vi "Chroma3.0.vi"() -> ()   [LabVIEW 2015]
uses:
  <vilib>/Utility/file.llb/Write To Spreadsheet File (string).vi
panel:
  in  "Run Name":string
  in  "Type (V_THD)":u32(ring) caption="Type (V_RMS)" items=["V_THD"=3, "V_PEAK-"=2, "V_RMS"=0, "V_PEAK+"=1]
  in  "Type (I_THD)":u32(ring) caption="Type (I_RMS)" items=["I_RMS"=0, "I_PEAK-"=2, "I_INRUSH"=3, "I_CRESTFACTOR"=4, "I_THD"=5, "I_PEAK+"=1]
  in  "Type (V_PEAK+)":u32(ring) caption="Type (V_RMS)" items=["V_THD"=3, "V_PEAK-"=2, "V_RMS"=0, "V_PEAK+"=1]
  in  "Type (P_FACTOR)":u32(ring) caption="Type (P_REAL)" items=["P_REAL"=0, "P_APPARENT"=1, "P_REACTIVE"=2, "P_ENERGY"=4, "P_FACTOR"=3]
  in  "Type (P_REACTIVE)":u32(ring) caption="Type (P_REAL)" items=["P_REAL"=0, "P_APPARENT"=1, "P_FACTOR"=3, "P_ENERGY"=4, "P_REACTIVE"=2]
  in  "Type (P_APPARENT)":u32(ring) caption="Type (P_REAL)" items=["P_ENERGY"=5, "P_FACTOR"=4, "P_REACTIVE"=2, "P_REAL"=0, "P_APPARENT"=1]
  in  "Type (I_CRESTFACTOR)":u32(ring) caption="Type (I_RMS)" items=["I_RMS"=0, "I_PEAK+"=1, "I_PEAK-"=2, "I_INRUSH"=3, "I_THD"=5, "I_CRESTFACTOR"=4]
  in  "Type (I_PEAK-)":u32(ring) caption="Type (I_RMS)" items=["I_RMS"=0, "I_PEAK+"=1, "I_INRUSH"=3, "I_CRESTFACTOR"=4, "I_THD"=5, "I_PEAK-"=2]
  in  "Type (I_PEAK+)":u32(ring) caption="Type (I_RMS)" items=["I_RMS"=0, "I_PEAK-"=2, "I_INRUSH"=3, "I_CRESTFACTOR"=4, "I_THD"=5, "I_PEAK+"=1]
  in  "Type (V_PEAK-)":u32(ring) caption="Type (V_RMS)" items=["V_RMS"=0, "V_PEAK+"=1, "V_THD"=3, "V_PEAK-"=2]
  out "Current Data Point Count":i32
  in  "STOP":bool
  in  "Type (V_RMS)":u32(ring) items=["V_THD"=3, "V_PEAK-"=2, "V_PEAK+"=1, "V_RMS"=0]
  in  "Type (I_RMS)":u32(ring) items=["I_THD"=5, "I_CRESTFACTOR"=4, "I_INRUSH"=3, "I_PEAK-"=2, "I_PEAK+"=1, "I_RMS"=0]
  in  "Type (P_REAL)":u32(ring) items=["P_ENERGY"=4, "P_FACTOR"=3, "P_REACTIVE"=2, "P_APPARENT"=1, "P_REAL"=0]
  in  "Port Name":refnum<k15> caption="resource name"
  in  "Minutes per test":dbl
  in  "Name of File":string
  in  "HOW MANY TEST":i32
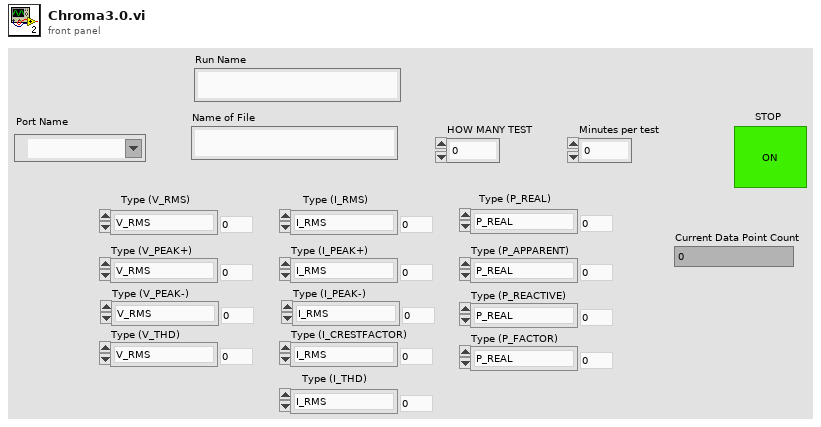
[diagram p1: front panel]
types:
  T1 = enum16{"open", "replace", "create", "open or create", "replace or create", "replace or create with confirmation"}
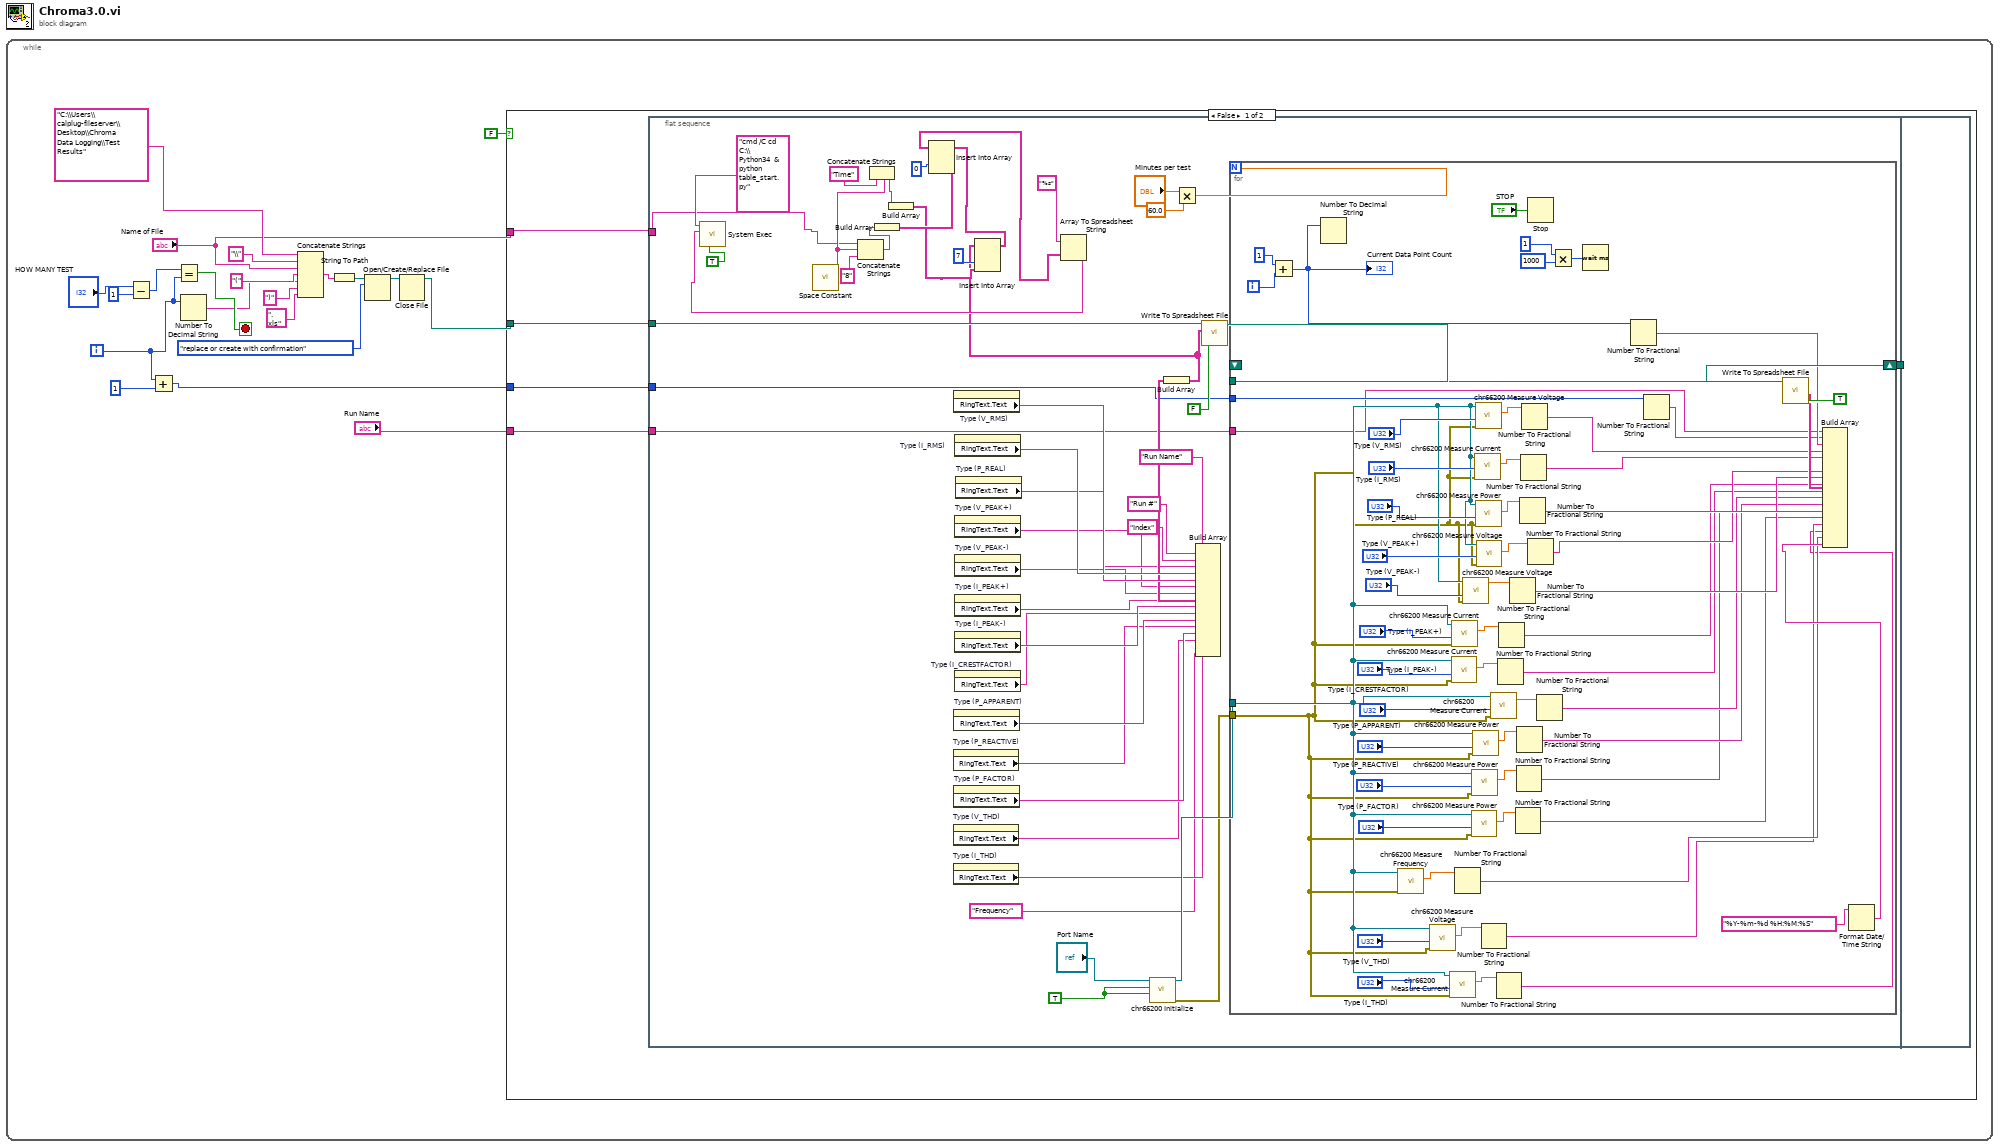
[diagram p0: block diagram]
diagram:
  n1 = while {
    i -> [w4]
    stop <- w15 stop-if-true
    n2 = Subtract(x="HOW MANY TEST", y=1) -> (x-y=w12:i32)
    n3 = Add(x=w4, y=1 ("x")) -> (x+y=w2:i32)
    n4 = Equal?(x=w12, y=w4) -> (x = y?=w15:bool)
    n5 = Number To Decimal String(number=w4) -> (decimal integer string=w7:string)  [unwired: 1 in]
    n6 = Concatenate Strings("C:\\Users\\calplug-fileserver\\Desktop\\Chroma Data Logging\\Test Results" ("string"), "\\" ("string"), "Name of File", "(" ("string"), w7, ")" ("string"), ".xls" ("string")) -> (w18:string)
    n7 = String To Path(string=w18) -> (path=w19:path)
    n8 = Open/Create/Replace File(file path (use dialog)=w19, operation (0:open)=T1."replace or create with confirmation") -> (refnum out=w17:refnum<file>)  [unwired: 4 in, 2 out]
    n9 = Close File(refnum=w17) -> (path=w16:path)  [unwired: 1 in, 1 out]
    n10 = case shown="False" FALSE {
      tunnel: w16 -> [w26 _]
      tunnel: "Name of File" -> [w24 _]
      tunnel: w2 -> [w23 _]
      tunnel: "Run Name" -> [w22 _]
      frame False {
        n11 = flat-sequence {
          tunnel: w26 -> [w73]
          tunnel: [w74] -> w25
          tunnel: w24 -> [w55]
          tunnel: w23 -> [w31]
          tunnel: w22 -> [w27]
          tunnel: w25 -> [_]
          frame #0 {
            w46 = TRUE
            n12 = call <vilib>:"Space Constant.vi"() -> ("String"=w60:string)
            n13 = Concatenate Strings(w55, w60, "8") -> (w62:string)
            n14 = Concatenate Strings("Time", w60) -> (w57:string)
            n15 = Build Array(w62) -> (w63:string[])
            n16 = Build Array(w57) -> (w58:string[])
            n17 = property on="Type (P_REACTIVE)" class="Ring (strict)"() -> ("RingText.Text"=w35:string)  [unwired: 2 in, 2 out]
            n18 = property on="Type (V_THD)" class="Ring (strict)"() -> ("RingText.Text"=w34:string)  [unwired: 2 in, 2 out]
            n19 = property on="Type (I_THD)" class="Ring (strict)"() -> ("RingText.Text"=w33:string)  [unwired: 2 in, 2 out]
            n20 = property on="Type (V_RMS)" class="Ring (strict)"() -> ("RingText.Text"=w48:string)  [unwired: 2 in, 2 out]
            n21 = property on="Type (P_APPARENT)" class="Ring (strict)"() -> ("RingText.Text"=w37:string)  [unwired: 2 in, 2 out]
            n22 = property on="Type (P_FACTOR)" class="Ring (strict)"() -> ("RingText.Text"=w36:string)  [unwired: 2 in, 2 out]
            n23 = property on="Type (I_RMS)" class="Ring (strict)"() -> ("RingText.Text"=w52:string)  [unwired: 2 in, 2 out]
            n24 = property on="Type (V_PEAK+)" class="Ring (strict)"() -> ("RingText.Text"=w42:string)  [unwired: 2 in, 2 out]
            n25 = property on="Type (V_PEAK-)" class="Ring (strict)"() -> ("RingText.Text"=w41:string)  [unwired: 2 in, 2 out]
            n26 = property on="Type (I_PEAK+)" class="Ring (strict)"() -> ("RingText.Text"=w40:string)  [unwired: 2 in, 2 out]
            n27 = property on="Type (I_PEAK-)" class="Ring (strict)"() -> ("RingText.Text"=w39:string)  [unwired: 2 in, 2 out]
            n28 = property on="Type (I_CRESTFACTOR)" class="Ring (strict)"() -> ("RingText.Text"=w38:string)  [unwired: 2 in, 2 out]
            n29 = property on="Type (P_REAL)" class="Ring (strict)"() -> ("RingText.Text"=w51:string)  [unwired: 2 in, 2 out]
            n30 = call <instrlib>:"chr66200 Initialize.vi"("Reset Device (Yes)"=w46, "ID Query (Yes)"=w46, "resource name"="Port Name") -> ("error out"=w43:errorcluster, "instrument handle out"=w44:refnum<k15>)  [unwired: 7 in]
            n31 = Multiply(x="Minutes per test", y=60.0) -> (x*y=w71:dbl)
            n32 = Build Array("Run Name", "Run #", "Index", w48, w52, w51, w42, w41, w40, w39, w38, w37, w35, w36, w34, w33, "Frequency") -> (w50:string[])
            n33 = Build Array(w50) -> (w49:string[][])
            n34 = Insert Into Array(array=w49, index (col)=7, new element=w58) -> (w65:string[][])  [unwired: 1 in]
            n35 = Insert Into Array(array=w65, index (col)=0, new element=w63) -> (w53:string[][])  [unwired: 1 in]
            n36 = Array To Spreadsheet String(array=w53, 3:"%s") -> (spreadsheet string=w54:string)  [unwired: 1 in]
            n37 = call <vilib>:"System Exec.vi"("run minimized? (F)"=TRUE, "standard input"=w54, "command line"="cmd /C cd C:\\Python34  & python table_start.py") -> ()  [unwired: 5 in, 4 out]
            n38 = call-poly <vilib>:"Write To Spreadsheet File.vi"("append to file? (new file:F)"=FALSE, "2D data"=w49, "file path (dialog if empty)"=w73) -> ("new file path (Not A Path if cancelled)"=w72:path)  [unwired: 5 in]
            n39 = for {
              N: w71 -> [_]
              tunnel: w72 -> [w131]
              shift-right: [w129] -> w74
              shift-left: _ -> [_]
              tunnel: w44 -> [w85]
              tunnel: w43 -> [w84]
              tunnel: w31 -> [w78]
              tunnel: w27 -> [w75]
              i -> [w80]
              n40 = Add(x=1, y=w80) -> (x+y=w76:i32)
              "Current Data Point Count" <- w76
              n41 = Number To Decimal String(number=w76) -> ()  [unwired: 1 in, 1 out]
              n42 = call <instrlib>:"chr66200 Measure Frequency.vi"("error in (no error)"=w84, "instrument handle"=w85) -> ("Read Value"=w101:dbl)  [unwired: 7 in, 2 out]
              n43 = call <instrlib>:"chr66200 Measure Voltage.vi"("error in (no error)"=w84, "Type (V_RMS)"="Type (V_THD)", "instrument handle"=w85) -> ("Read Value"=w87:dbl)  [unwired: 6 in, 2 out]
              n44 = call <instrlib>:"chr66200 Measure Current.vi"("error in (no error)"=w84, "Type (I_RMS)"="Type (I_THD)", "instrument handle"=w85) -> ("Read Value"=w90:dbl)  [unwired: 6 in, 2 out]
              n45 = call <instrlib>:"chr66200 Measure Current.vi"("error in (no error)"=w84, "Type (I_RMS)"="Type (I_PEAK-)", "instrument handle"=w85) -> ("Read Value"=w109:dbl)  [unwired: 6 in, 2 out]
              n46 = call <instrlib>:"chr66200 Measure Current.vi"("error in (no error)"=w84, "Type (I_RMS)"="Type (I_PEAK+)", "instrument handle"=w85) -> ("Read Value"=w111:dbl)  [unwired: 6 in, 2 out]
              n47 = Number To Fractional String(number=w101) -> (F-format string=w83:string)  [unwired: 3 in]
              n48 = call <instrlib>:"chr66200 Measure Voltage.vi"("error in (no error)"=w84, "Type (V_RMS)"="Type (V_PEAK-)", "instrument handle"=w85) -> ("Read Value"=w113:dbl)  [unwired: 6 in, 2 out]
              n49 = call <instrlib>:"chr66200 Measure Power.vi"("error in (no error)"=w84, "Type (P_REAL)"="Type (P_FACTOR)", "instrument handle"=w85) -> ("Read Value"=w102:dbl)  [unwired: 6 in, 2 out]
              n50 = call <instrlib>:"chr66200 Measure Power.vi"("error in (no error)"=w84, "Type (P_REAL)"="Type (P_REACTIVE)", "instrument handle"=w85) -> ("Read Value"=w103:dbl)  [unwired: 6 in, 2 out]
              n51 = call <instrlib>:"chr66200 Measure Power.vi"("error in (no error)"=w84, "Type (P_REAL)"="Type (P_APPARENT)", "instrument handle"=w85) -> ("Read Value"=w105:dbl)  [unwired: 6 in, 2 out]
              n52 = call <instrlib>:"chr66200 Measure Current.vi"("error in (no error)"=w84, "Type (I_RMS)"="Type (I_RMS)", "instrument handle"=w85) -> ("Read Value"=w122:dbl)  [unwired: 6 in, 2 out]
              n53 = call <instrlib>:"chr66200 Measure Voltage.vi"("error in (no error)"=w84, "Type (V_RMS)"="Type (V_RMS)", "instrument handle"=w85) -> ("Read Value"=w123:dbl)  [unwired: 6 in, 2 out]
              n54 = call <instrlib>:"chr66200 Measure Power.vi"("error in (no error)"=w84, "Type (P_REAL)"="Type (P_REAL)", "instrument handle"=w85) -> ("Read Value"=w121:dbl)  [unwired: 6 in, 2 out]
              n55 = call <instrlib>:"chr66200 Measure Voltage.vi"("error in (no error)"=w84, "Type (V_RMS)"="Type (V_PEAK+)", "instrument handle"=w85) -> ("Read Value"=w116:dbl)  [unwired: 6 in, 2 out]
              n56 = Number To Fractional String(number=w87) -> (F-format string=w82:string)  [unwired: 3 in]
              n57 = call <instrlib>:"chr66200 Measure Current.vi"("error in (no error)"=w84, "Type (I_RMS)"="Type (I_CRESTFACTOR)", "instrument handle"=w85) -> ("Read Value"=w107:dbl)  [unwired: 6 in, 2 out]
              n58 = Number To Fractional String(number=w90) -> (F-format string=w81:string)  [unwired: 3 in]
              n59 = Number To Fractional String(number=w109) -> (F-format string=w108:string)  [unwired: 3 in]
              n60 = Number To Fractional String(number=w111) -> (F-format string=w110:string)  [unwired: 3 in]
              n61 = Number To Fractional String(number=w113) -> (F-format string=w112:string)  [unwired: 3 in]
              n62 = Number To Fractional String(number=w102) -> (F-format string=w92:string)  [unwired: 3 in]
              n63 = Number To Fractional String(number=w103) -> (F-format string=w93:string)  [unwired: 3 in]
              n64 = Number To Fractional String(number=w105) -> (F-format string=w104:string)  [unwired: 3 in]
              n65 = Number To Fractional String(number=w121) -> (F-format string=w117:string)  [unwired: 3 in]
              n66 = Number To Fractional String(number=w122) -> (F-format string=w118:string)  [unwired: 3 in]
              n67 = Number To Fractional String(number=w123) -> (F-format string=w119:string)  [unwired: 3 in]
              n68 = Stop(stop? (T)="STOP") -> ()
              n69 = Number To Fractional String(number=w116) -> (F-format string=w115:string)  [unwired: 3 in]
              n70 = Number To Fractional String(number=w107) -> (F-format string=w106:string)  [unwired: 3 in]
              n71 = Multiply(x=u32 1 ("Interval of Data Collection (sec)"), y=u32 1000) -> (x*y=w133:u32)
              n72 = Wait (ms)(milliseconds to wait=w133) -> ()  [unwired: 1 out]
              n73 = Number To Fractional String(number=w76) -> (F-format string=w79:string)  [unwired: 3 in]
              n74 = Number To Fractional String(number=w78) -> (F-format string=w77:string)  [unwired: 3 in]
              n75 = Format Date/Time String(time format string (%c)="%Y-%m-%d %H:%M:%S") -> (date/time string=w88:string)  [unwired: 2 in]
              n76 = Build Array(w75, w77, w79, w119, w118, w117, w115, w112, w110, w108, w106, w104, w93, w92, w82, w81, w83, w88) -> (w120:string[])
              n77 = call-poly <vilib>:"Write To Spreadsheet File.vi"("append to file? (new file:F)"=TRUE, "1D data"=w120, "file path (dialog if empty)"=w131) -> ("new file path (Not A Path if cancelled)"=w129:path)  [unwired: 5 in]
            }
          }
          frame #1 {
          }
        }
      }
      frame True {
      }
    }
  }
